vi "ASI Set ID.vi"(11 "iCameraID":i32) -> (3 "function return":i32)   [LabVIEW 2012, in "ASICamera2_no_err.lvlib"]
doc: "ASICAMERA_API ASI_ERROR_CODE ASISetID(int iCameraID, ASI_ID ID);"
uses:
  <userlib>/ASICamera2_no_err/ASICamera2_no_err.lvlib
  ASICamera2.dll
panel:
  in  "cluster":cluster{"id":dbl[]}
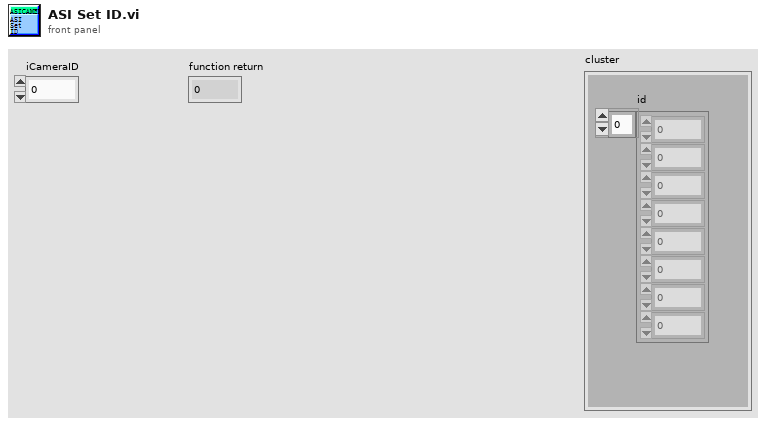
[diagram p1: front panel]
types:
  T1 = cluster{"id[0]":dbl, "id[1]":dbl, "id[2]":dbl, "id[3]":dbl, "id[4]":dbl, "id[5]":dbl, "id[6]":dbl, "id[7]":dbl, "id[8]":dbl}
  T2 = cluster{"id":cluster{"id[0]":dbl, "id[1]":dbl, "id[2]":dbl, "id[3]":dbl, "id[4]":dbl, "id[5]":dbl, "id[6]":dbl, "id[7]":dbl, "id[8]":dbl}}
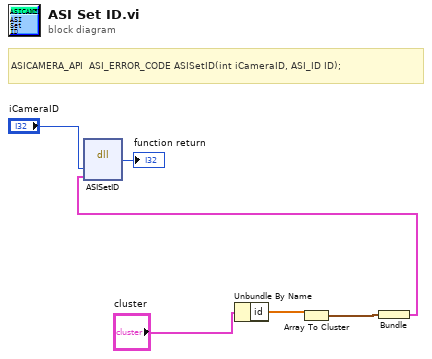
[diagram p0: block diagram]
diagram:
  # "ASICAMERA_API  ASI_ERROR_CODE ASISetID(int iCameraID, ASI_ID ID);"
  n1 = Unbundle By Name("cluster") -> ("id"=w3:dbl[])
  n2 = Array To Cluster(array=w3) -> (cluster=w2:T1)
  n3 = Bundle("id"=w2) -> (w1:T2)  [unwired: 1 in]
  n4 = dll-call lib="ASICamera2.*" fn="ASISetID"("iCameraID"="iCameraID", "id"=w1) -> ("返回类型"=→"function return":i32)  [unwired: 5 in, 2 out]
